vi "Get Logging Source.vi"() -> (3 "Logging Source":string)   [LabVIEW 2020, in "NI_SystemLogging.lvlib"]
uses:
  <vilib>/Utility/SystemLogging/NI_SystemLogging.lvlib
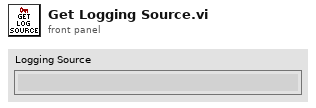
[diagram p1: front panel]
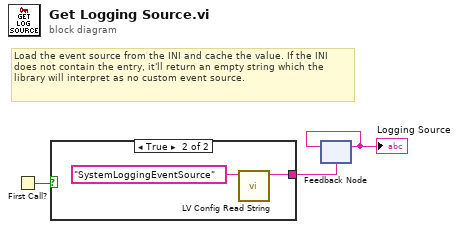
[diagram p0: block diagram]
diagram:
  # "Load the event source from the INI and cache the value. If the INI does not contain the entry, it'll return an empty string which the library will interpret as no custom event source."
  n1 = First Call?() -> (First Call?: T/F=w3:bool)
  n2 = case shown="True" w3 {
    tunnel: [_ w4] -> w2
    frame False {
    }
    frame True {
      n3 = call <resource>:"LV Config Read String.vi"("key"="SystemLoggingEventSource") -> ("value"=w4:string)  [unwired: 4 in, 2 out]
    }
  }
  n4 = feedback #1(w2) -> (w1:string)
  "Logging Source" <- w1
  n5 = feedback-in #1(w1) -> ()
